vi "Release.vi"(11 "Transport in":refnum<class "Transport.lvclass">) -> (2 "Unhandled Msgs":refnum<class "Msg.lvclass">[](array[class]))   [LabVIEW 2025, in "jettl.lvlib" / "Transport.lvlib" / "Transport.lvclass"]
uses:
  Transport.lvclass
  Msg/Msg.lvclass
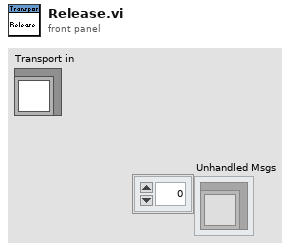
[diagram p1: front panel]
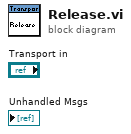
[diagram p0: block diagram]
diagram:
